vi "RTM SLSC Export.vi"(8 "error in (no error)":errorcluster, 11 "Node Ptr":T1=18446744073709551615 format="%.0x") -> (0 "error out":errorcluster)   [LabVIEW 2020, in "SLSC EDS System Explorer.lvlib"]
uses:
  SLSC EDS System Explorer.lvlib
  <vilib>/NI VeriStand/Custom Device API/Custom Device Item Ref.ctl
  Shared/Constants.vi
  SLSC CD API/SLSC CD System Explorer/SLSC CD System Explorer.lvlib
  Shared/SLSC EDS Shared.lvlib
  <vilib>/NI VeriStand/Custom Device API/Custom Device API.lvlib
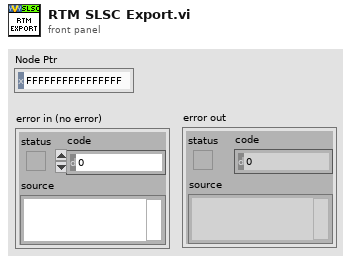
[diagram p1: front panel]
types:
  T1 = typedef "Custom Device API.lvlib/Custom Device Item Ref.ctl" = u64
  T2 = typedef "EDSjsonStructure.ctl" = cluster{"vendorNum":u32, "vendorName":string, "vendorPrefix":string, "productNum":u32, "productName":string, "capsVersion":string, "capsSpecVersion":u32, "capsSpecOldestCompatibleVersion":u32, "enums":T3[], "properties":T4[], "commands":T5[], "scales":T6[], "physicalChannels":T7[], "registerMap":cluster{"registers":T8[]}}
  T3 = typedef "enum.ctl" = cluster{"name":string, "description-en":string, "values":cluster{"name":string, "description-en":string, "value":i32}[]}
  T4 = typedef "property.ctl" = cluster{"name":string, "description-en":string, "documentation-en":string, "dataType":string, "bitfield":string, "access":string, "scale":string, "value":variant, "min":variant, "max":variant, "default value":variant}
  T5 = typedef "command.ctl" = cluster{"name":string, "description-en":string, "documentation-en":string, "startBitfield":string, "waitTimeInMs":i32, "doneBitfield":string, "doneInterrupt":string, "doneTimeoutInMs":i32, "value":variant}
  T6 = typedef "scale.ctl" = cluster{"name":string, "description-en":string, "m":dbl, "b":dbl, "forwardCoeffs":dbl[], "reverseCoeffs":dbl[], "coercion":string, "table":cluster{"scaled":dbl, "unscaled":dbl}[]}
  T7 = typedef "physicalChannel.ctl" = cluster{"name":string, "description-en":string, "commands":T5[], "properties":T4[]}
  T8 = typedef "register.ctl" = cluster{"name":string, "description-en":string, "access":string, "address":u32, "size":u32, "bitfields":cluster{"name":string, "description-en":string, "offset":u32, "size":u32, "signed":bool, "strobe":bool}[]}
  T9 = typedef "Custom Device API.lvlib/Custom Device Item Info.ctl" = cluster{"Name":string, "Is Channel":bool, "GUID":string, "Is Waveform":bool}
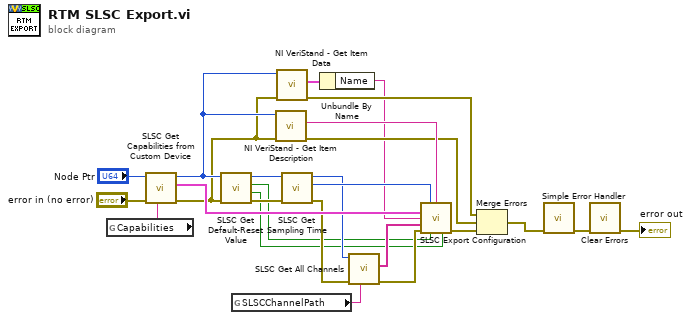
[diagram p0: block diagram]
diagram:
  n1 = global read "Constants.vi" "Capabilities"() -> (w25:string)
  n2 = call "SLSC Get Capabilities from Custom Device.vi"("Property Name"=w25, "error in (no error)"="error in (no error)", "Device Item Ref in"="Node Ptr") -> ("error out"=w1:errorcluster, "data"=w16:T2, "Item Ref out"=w7:T1)  [unwired: 3 in, 3 out]
  n3 = call "SLSC Get Default-Reset Value.vi"("error in (no error)"=w1, "Section Ref in"=w7) -> ("error out"=w12:errorcluster, "Apply Reset"=w10:bool, "Apply Default"=w9:bool, "Item Ref out"=w11:T1)  [unwired: 6 in]
  n4 = global read "Constants.vi" "SLSCChannelPath"() -> (w20:string)
  n5 = call <vilib>:"NI VeriStand - Get Item Description.vi"("error in (no error)"=w1, "Item Ref in"=w7) -> ("error out"=w3:errorcluster, "Description"=w6:string)  [unwired: 6 in, 2 out]
  n6 = call <vilib>:"NI VeriStand - Get Item Data.vi"("error in (no error)"=w1, "Item Ref in"=w7) -> ("error out"=w4:errorcluster, "Item Info"=w8:T9)  [unwired: 8 out]
  n7 = call "SLSC Get Sampling Time.vi"("error in (no error)"=w12, "Item Ref in"=w11) -> ("error out"=w13:errorcluster, "Loop time (ms)"=w15:u32, "Section Ref out"=w14:T1)  [unwired: 7 in]
  n8 = Unbundle By Name(w8) -> ("Name"=w2:string)
  n9 = call "SLSC Get All Channels.vi"("SLSCChannelPath"=w20, "error in (no error)"=w13, "Item Ref in"=w14) -> ("error out"=w18:errorcluster, "TreeItem Channels"=w19:string[])  [unwired: 5 in, 2 out]
  n10 = call "SLSC Export Configuration.vi"("Loop rate"=w15, "Description"=w6, "SLSC EDS module in"=w16, "Custom Device Name"=w2, "Channels to Enable"=w19, "error in (no error)"=w18, "Apply Default"=w9, "Apply Reset"=w10) -> ("error out"=w17:errorcluster)  [unwired: 7 in]
  n11 = Merge Errors(w4, w3, w17) -> (w5:errorcluster)
  n12 = call <vilib>:"Simple Error Handler.vi"("error in (no error)"=w5) -> ("error out"=w22:errorcluster)  [unwired: 4 in, 4 out]
  n13 = call <vilib>:"Clear Errors.vi"("error in (no error)"=w22) -> ("error out"=→"error out":errorcluster)  [unwired: 5 in, 1 out]
